vi "Stop Core.vi"(10 "final error code":i32, 11 "Network Stream in":refnum<class "Network Stream.lvclass">) -> (3 "Network Stream out":refnum<class "Network Stream.lvclass">)   [LabVIEW 2014, in "Network Stream.lvlib" / "Network Stream.lvclass"]
doc: "(<B>Filename</B>: Actor Framework.lvlib:Actor.lvclass:Stop Core.vi)\n\nDefines what the actor does before it stops. Use the <B>final error code</B> input to determine whether the actor shut down in response to an error.\n\nBy default, this method does nothing. A descendant class may override it to define behavior, such as shutting down any processes the actor initiated in its override of the Actor Core method."
uses:
  Network Stream.lvclass
  Proxy/Proxy/Proxy.lvclass
panel:
  # "PROXY ACTOR\n HAS STOPED"
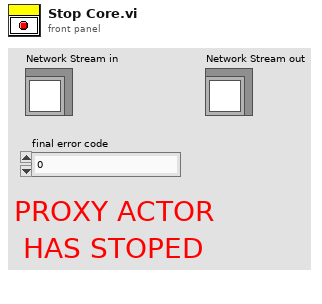
[diagram p1: front panel]
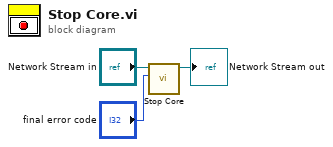
[diagram p0: block diagram]
diagram:
  n1 = call-parent "Stop Core.vi"("final error code"="final error code", "Proxy in"="Network Stream in") -> ("Proxy out"=→"Network Stream out":refnum<class "Network Stream.lvclass">)  [unwired: 9 in]
